vi "Start Test.vi"(10 "Tests":string[](array[string]), 11 "Result Model In":refnum<class "Result Model.lvclass">) -> (3 "Result Model Out":refnum<class "Result Model.lvclass">)   [LabVIEW 2020, in "Result Model.lvclass"]
uses:
  Result Model.lvclass
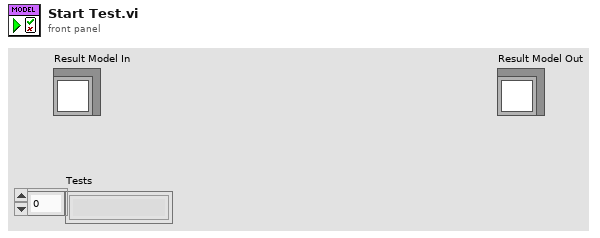
[diagram p1: front panel]
types:
  T1 = typedef "Result.lvlib/Status.ctl" = enum16{"", "Passed", "Failed", "Error", "Skipped", "Setup Error", "Broken", "Teardown Error"}
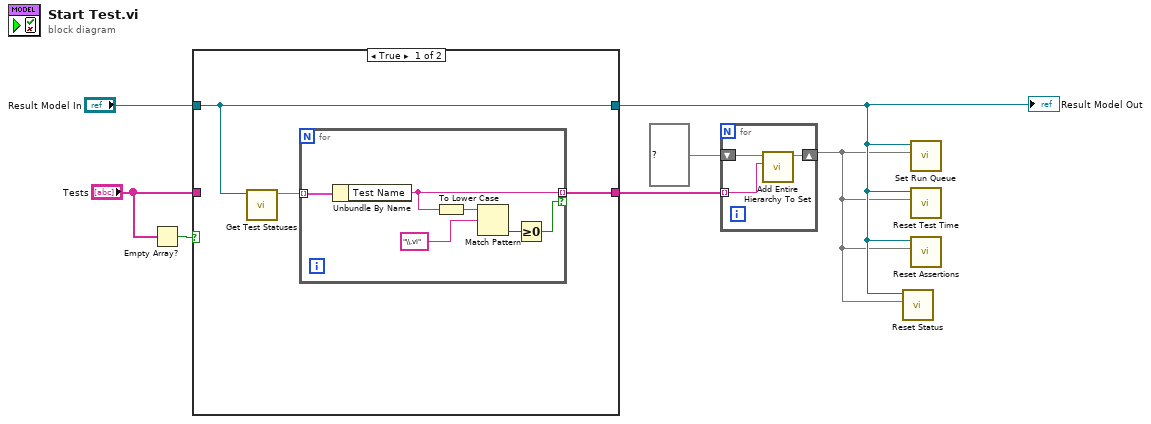
[diagram p0: block diagram]
diagram:
  n1 = Empty Array?(array="Tests") -> (empty?=w6:bool)
  n2 = case shown="True" w6 {
    tunnel: "Result Model In" -> [w9 w18]
    tunnel: [w9 w18] -> w2
    tunnel: "Tests" -> [_ w17]
    tunnel: [w8 w17] -> w3
    frame True {
      n3 = call "Get Test Statuses.vi"("Result Model in"=w9) -> ("Test Statuses"=w10:map{string, T1})  [unwired: 10 in]
      n4 = for {
        tunnel: w10 -> [w16] mode=indexing
        tunnel: [w12] -> w8 mode=indexing if=w11
        n5 = Unbundle By Name(w16) -> ("Test Name"=w12:string)
        n6 = To Lower Case(string=w12) -> (all lower case string=w13:string)
        n7 = Match Pattern(string=w13, regular expression="\\.vi") -> (offset past match=w14:i32)  [unwired: 1 in, 3 out]
        n8 = Greater Or Equal To 0?(x=w14) -> (x >= 0?=w11:bool)
      }
    }
    frame False {
    }
  }
  "Result Model Out" <- w2
  n9 = for {
    shift-right: [w20] -> w1
    shift-left: set{string} {} ("Run Queue") -> [w21]
    tunnel: w3 -> [w19] mode=indexing
    n10 = call "Add Entire Hierarchy To Set.vi"("Test Name"=w19, "Set in"=w21) -> ("Set out"=w20:set{string})  [unwired: 9 in]
  }
  n11 = call "Reset Status.vi"("Run Queue"=w1, "Result Model in"=w2) -> ()  [unwired: 10 in]
  n12 = call "Set Run Queue.vi"("Run Queue"=w1, "Result Model in"=w2) -> ()  [unwired: 10 in]
  n13 = call "Reset Test Time.vi"("Run Queue"=w1, "Result Model in"=w2) -> ()  [unwired: 10 in]
  n14 = call "Reset Assertions.vi"("Run Queue"=w1, "Result Model in"=w2) -> ()  [unwired: 10 in]
